vi "Progress Dialog CORE.vi"(11 "Progress Dialog in":refnum<class "Progress Dialog.lvclass">) -> ()   [LabVIEW 2011, in "COSYLib.lvlib" / "Progress Dialog.lvclass"]
uses:
  Progress Dialog.lvclass
  Progress dialog type.ctl
  <vilib>/Utility/miscctls.llb/LVPointTypeDef.ctl
  Progress Dialog.lvclass/Progress Dialog.ctl
panel:
  out "Ring":u16(ring)
  in  "Stop":bool
  out "Cancelled?":bool
  in  "Cancel":bool
  out "Text":string
  out "Progress":dbl(slide) scale=0.0..100.0
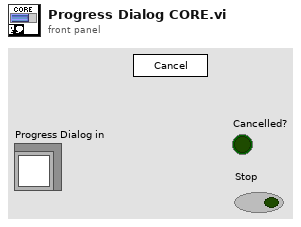
[diagram p1: front panel]
types:
  T1 = typedef "COSYLib.lvlib/Progress Dialog.lvclass/Progress dialog type.ctl" = enum16{"Progress", "Marquee"}
  T2 = typedef "LVPointTypeDef.ctl" = cluster{"Horizontal":i16, "Vertical":i16}
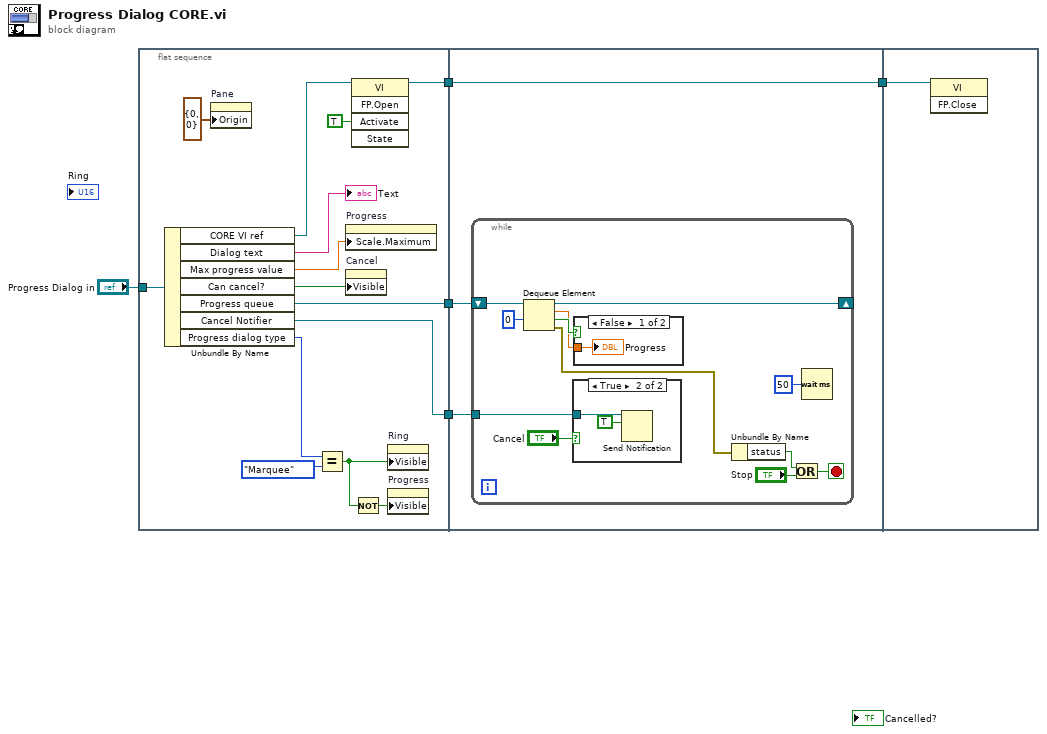
[diagram p0: block diagram]
diagram:
  n1 = flat-sequence {
    tunnel: "Progress Dialog in" -> [w18]
    tunnel: [w17] -> w4
    tunnel: [w16] -> w3
    tunnel: [w10] -> w1
    tunnel: w4 -> [w22]
    tunnel: w3 -> [w21]
    tunnel: [w20] -> w2
    tunnel: w1 -> [w20]
    tunnel: w2 -> [w38]
    frame #0 {
      n2 = Unbundle By Name(w18) -> ("CORE VI ref"=w11:refnum<vi>, "Dialog text"=→"Text":string, "Max progress value"=w12:dbl, "Can cancel?"=w15:bool, "Progress queue"=w17:refnum<queue>, "Cancel Notifier"=w16:refnum<notifier>, "Progress dialog type"=w9:T1)
      n3 = property on="Pane" class="Pane"("Origin"=T2 {"Horizontal"=0, "Vertical"=0}) -> ()  [unwired: 2 in, 2 out]
      n4 = Equal?(x=w9, y=Progress_dialog_type."Marquee") -> (x = y?=w6:bool)
      n5 = property on="Progress" class="Slide (strict)"("Scale.Maximum"=w12) -> ()  [unwired: 2 in, 2 out]
      n6 = property on="Cancel" class="Bool"("Visible"=w15) -> ()  [unwired: 2 in, 2 out]
      n7 = invoke class="VI" method="FP.Open"(reference=w11, "Activate"=TRUE ("Activate?")) -> (reference out=w10:refnum<vi>)  [unwired: 3 in, 4 out]
      n8 = Not(x=w6) -> (.not. x?=w7:bool)
      n9 = property on="Ring" class="Ring (strict)"("Visible"=w6) -> ()  [unwired: 2 in, 2 out]
      n10 = property on="Progress" class="Slide (strict)"("Visible"=w7) -> ()  [unwired: 2 in, 2 out]
    }
    frame #1 {
      n11 = while {
        shift-right: [w29] -> _
        shift-left: w22 -> [w32]
        tunnel: w21 -> [w26]
        stop <- w25 stop-if-true
        n12 = Dequeue Element(queue=w32, timeout in ms (-1)=0) -> (queue out=w29:refnum<queue>, element=w28:dbl, timed out?=w30:bool, error out=w23:errorcluster)  [unwired: 1 in]
        n13 = case shown="True" "Cancel" {
          tunnel: w26 -> [_ w36]
          frame False {
          }
          frame True {
            n14 = Send Notification(notification=TRUE, notifier=w36) -> ()  [unwired: 1 in, 2 out]
          }
        }
        n15 = case shown="False" w30 {
          tunnel: w28 -> [w37 _]
          frame False {
            "Progress" <- w37
          }
          frame True {
          }
        }
        n16 = Unbundle By Name(w23) -> ("status"=w24:bool)
        n17 = Or(x=w24, y="Stop") -> (x .or. y?=w25:bool)
        n18 = Wait (ms)(milliseconds to wait=u32 50) -> ()  [unwired: 1 out]
      }
    }
    frame #2 {
      n19 = invoke class="VI" method="FP.Close"(reference=w38) -> ()  [unwired: 2 in, 3 out]
    }
  }
